vi "2_SLMs.vi"() -> ()   [LabVIEW 2010]
panel:
  in  "R2":dbl(slide) scale=0.0..1.0
  in  "G2":dbl(slide) scale=0.0..1.0
  in  "B2":dbl(slide) scale=0.0..1.0
  out "packet sent to SLM 2":string
  out "packet sent to SLM 1":string
  in  "B1":dbl(slide) scale=0.0..1.0
  in  "G1":dbl(slide) scale=0.0..1.0
  in  "R1":dbl(slide) scale=0.0..1.0
  in  "stop":bool
  # "This is a very simple demo showing how to use two copies of the hologram engine to address two SLMs."
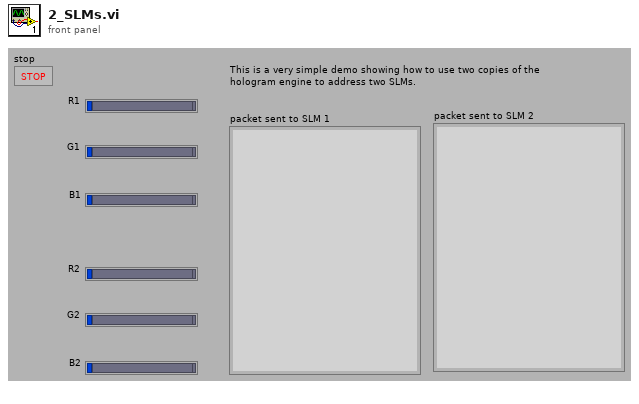
[diagram p1: front panel]
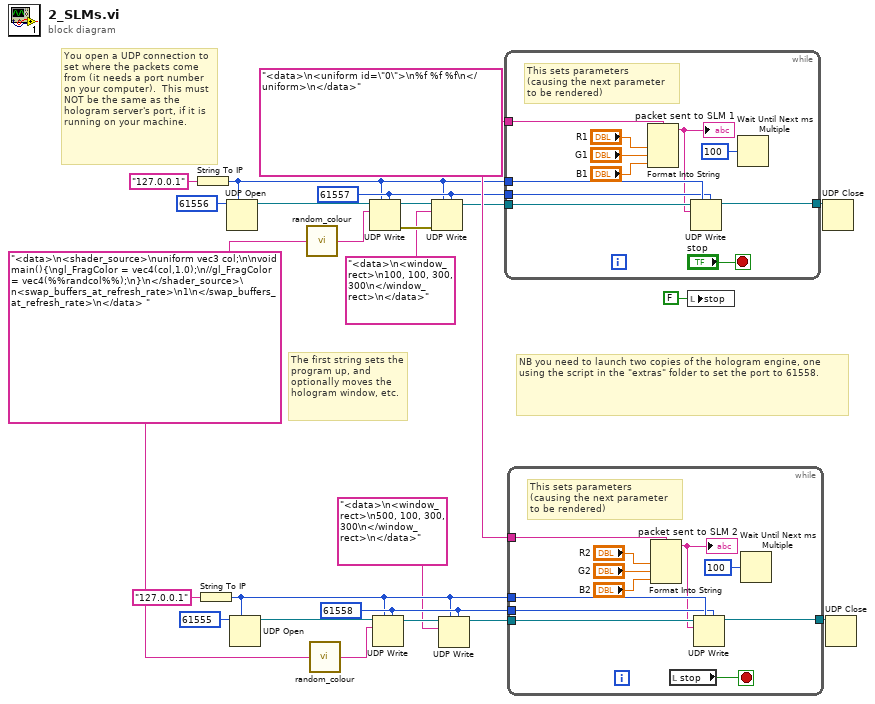
[diagram p0: block diagram]
diagram:
  w3 = u16 61558 ("port")
  w13 = "<data>\n<uniform id=\"0\">\n%f %f %f\n</uniform>\n</data>" ("data in")
  w14 = "<data>\n<shader_source>\nuniform vec3 col;\n\nvoid main(){\ngl_FragColor = vec4(col,1.0);\n//gl_FragColor = vec4(%%randcol%%);\n}\n</shader_source>\n<swap_buffers_at_refresh_rate>\n1\n</swap_buffers_at_refresh_rate>\n</data> " ("data in")
  w8 = u16 61557 ("port")
  # "NB you need to launch two copies of the hologram engine, one using the script in the \"extras\" folder to set the port to 61558."
  # "You open a UDP connection to set where the packets come from (it needs a port number on your computer).  This must NOT be the same as the hologram server's port, if it is running on your machine."
  # "The first string sets the program up, and optionally moves the hologram window, etc."
  n1 = String To IP(1:"127.0.0.1" ("name")) -> (0:w7:u32)
  n2 = String To IP(1:"127.0.0.1" ("name")) -> (0:w2:u32)
  n3 = UDP Open(7:w7, 11:u16 61556 ("port")) -> (port=w24:refnum<k16>)  [unwired: 3 in, 2 out]
  n4 = UDP Open(7:w2, 11:u16 61555 ("port")) -> (port=w15:refnum<k16>)  [unwired: 3 in, 2 out]
  n5 = call "random_colour.vi"("string in"=w14) -> ("string out, with %%randcol%% replaced with a 4-element colour"=w20:string)
  n6 = call "random_colour.vi"("string in"=w14) -> ("string out, with %%randcol%% replaced with a 4-element colour"=w19:string)
  n7 = UDP Write(address=w7, port or service name=w8, connection ID=w24, data in=w20) -> (error out=w11:errorcluster, 3:w10:refnum<k16>)  [unwired: 2 in]
  n8 = UDP Write(address=w2, port or service name=w3, connection ID=w15, data in=w19) -> (3:w4:refnum<k16>)  [unwired: 2 in, 1 out]
  n9 = UDP Write(address=w7, port or service name=w8, connection ID=w10, data in="<data>\n<window_rect>\n100, 100, 300, 300\n</window_rect>\n</data>", 8:w11) -> (3:w9:refnum<k16>)  [unwired: 1 in, 1 out]
  n10 = UDP Write(address=w2, port or service name=w3, connection ID=w4, data in="<data>\n<window_rect>\n500, 100, 300, 300\n</window_rect>\n</data>") -> (3:w5:refnum<k16>)  [unwired: 2 in, 1 out]
  n11 = while {
    tunnel: w9 -> [w35]
    tunnel: [w34] -> w22
    tunnel: w7 -> [w33]
    tunnel: w8 -> [w32]
    tunnel: w13 -> [w31]
    stop <- "stop" stop-if-true
    # "This sets parameters\n(causing the next parameter\nto be rendered)"
    n12 = Format Into String(format string=w31, "R1", "G1", "B1") -> (resulting string=w30:string)  [unwired: 2 in, 1 out]
    "packet sent to SLM 1" <- w30
    n13 = UDP Write(address=w33, port or service name=w32, connection ID=w35, data in=w30) -> (3:w34:refnum<k16>)  [unwired: 2 in, 1 out]
    n14 = Wait Until Next ms Multiple(millisecond multiple=u32 100) -> ()  [unwired: 1 out]
  }
  n15 = while {
    tunnel: w5 -> [w46]
    tunnel: [w45] -> w17
    tunnel: w2 -> [w44]
    tunnel: w3 -> [w43]
    tunnel: w13 -> [w42]
    stop <- w36 stop-if-true
    # "This sets parameters\n(causing the next parameter\nto be rendered)"
    n16 = Format Into String(format string=w42, "R2", "G2", "B2") -> (resulting string=w41:string)  [unwired: 2 in, 1 out]
    "packet sent to SLM 2" <- w41
    n17 = local read "stop"() -> (w36:bool)
    n18 = UDP Write(address=w44, port or service name=w43, connection ID=w46, data in=w41) -> (3:w45:refnum<k16>)  [unwired: 2 in, 1 out]
    n19 = Wait Until Next ms Multiple(millisecond multiple=u32 100) -> ()  [unwired: 1 out]
  }
  n20 = local write "stop"(FALSE ("stop")) -> ()
  n21 = UDP Close(connection ID=w22) -> ()  [unwired: 1 in, 2 out]
  n22 = UDP Close(connection ID=w17) -> ()  [unwired: 1 in, 2 out]
